vi "ImportExcelValues.vi"(8 "error in (no error)":errorcluster, 9 "List In":refnum<class "List.lvclass">, 10 "ExcelPath":path, 11 "Excel in":refnum<class "Excel.lvclass">) -> (0 "error out":errorcluster, 2 "Sheets":refnum<class "List.lvclass">[](array[class]), 3 "Excel out":refnum<class "Excel.lvclass">)   [LabVIEW 2015, in "Excel.lvclass"]
uses:
  Excel.lvclass
  _list/List.lvclass
  Excel.lvclass/Excel.ctl
  Read_Excel_Values.llb/GetXL_CellValues_2D_String.vi
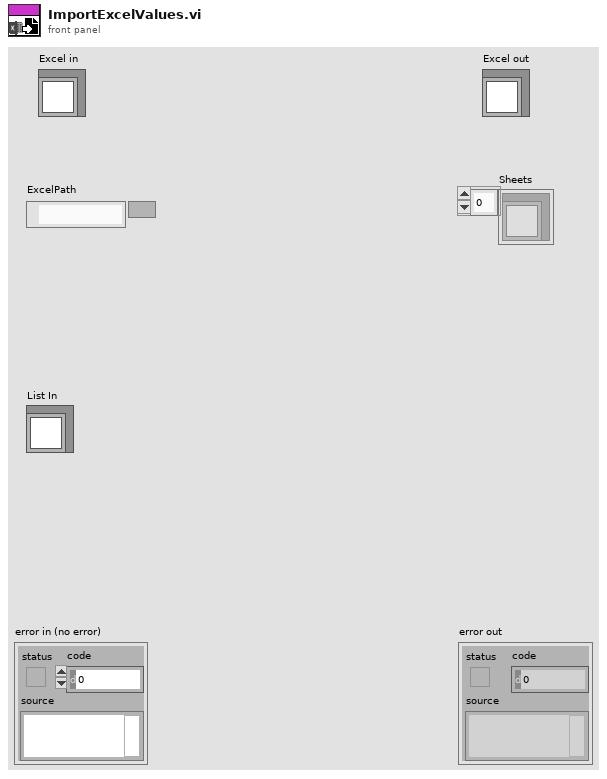
[diagram p1: front panel]
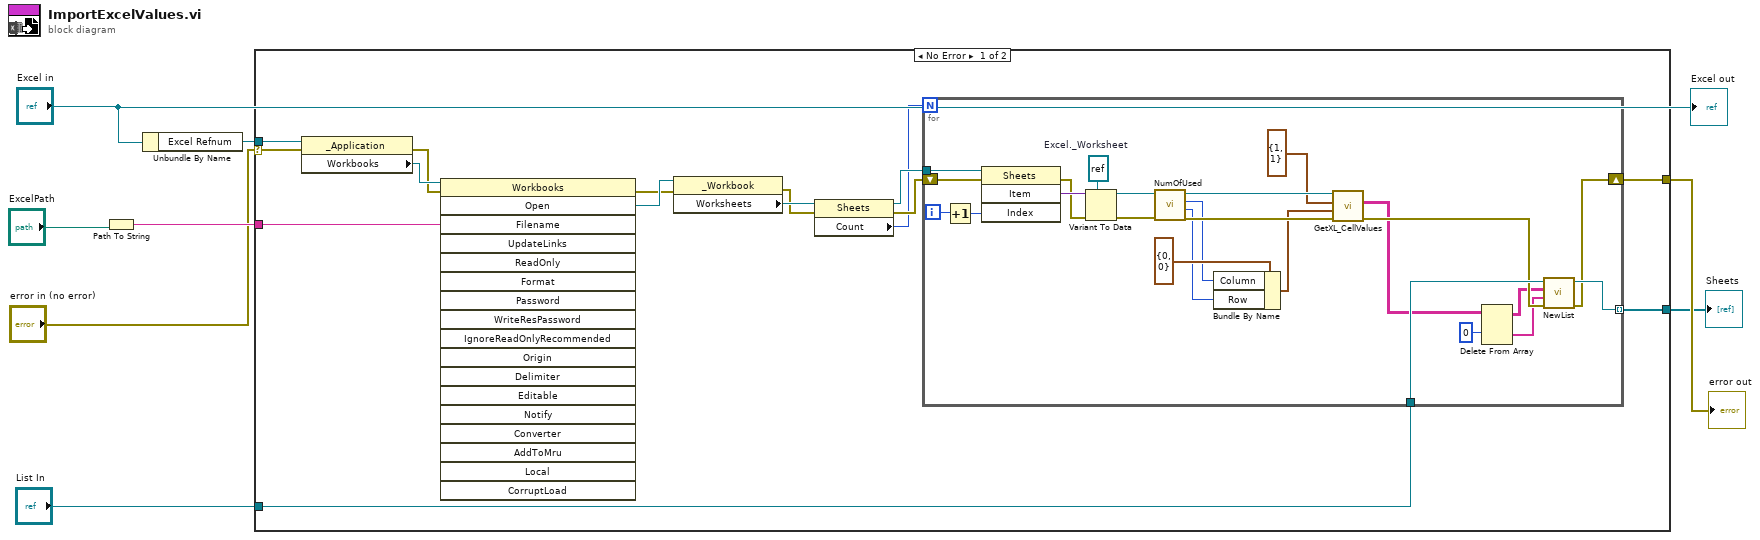
[diagram p0: block diagram]
diagram:
  n1 = Path To String(path="ExcelPath") -> (string=w6:string)
  n2 = Unbundle By Name("Excel in") -> ("Excel Refnum"=w8:refnum<k7>)
  n3 = case shown="No Error" "error in (no error)" {
    selector: "error in (no error)" -> [w16 w48]
    tunnel: w8 -> [w23 _]
    tunnel: w6 -> [w21 _]
    tunnel: [w11 w48] -> w5
    tunnel: [w10 _] -> w2
    tunnel: "List In" -> [w9 _]
    frame No Error {
      n4 = property class="_Application"(reference=w23, error in=w16) -> (error out=w15:errorcluster, "Workbooks"=w22:refnum<k7>)  [unwired: 1 out]
      n5 = invoke class="Workbooks" method="Open"(reference=w22, error in=w15, "Filename"=w21) -> (error out=w14:errorcluster, "Open"=w20:refnum<k7>)  [unwired: 15 in, 16 out]
      n6 = property class="_Workbook"(reference=w20, error in=w14) -> (error out=w13:errorcluster, "Worksheets"=w19:refnum<k7>)  [unwired: 1 out]
      n7 = property class="Sheets"(reference=w19, error in=w13) -> (reference out=w18:refnum<k7>, error out=w17:errorcluster, "Count"=w12:i32)
      n8 = for {
        N: w12 -> [_]
        tunnel: w18 -> [w47]
        shift-right: [w24] -> w11
        shift-left: w17 -> [w46]
        tunnel: [w25] -> w10 mode=indexing
        tunnel: w9 -> [w30]
        i -> [w33]
        w45 = refnum<k7> refnum  # Excel._Worksheet
        n9 = Increment(x=w33) -> (x+1=w32:i32)
        n10 = invoke class="Sheets" method="Item"(reference=w47, error in=w46, "Index"=w32) -> (error out=w34:errorcluster, "Item"=w44:variant)  [unwired: 1 in, 2 out]
        n11 = Variant To Data(error in=w34, type=w45, Variant=w44) -> (data=w43:refnum<k7>, error out=w42:errorcluster)
        n12 = call "NumOfUsed.vi"("error in (no error)"=w42, "worksheet_Refnum"=w43) -> ("error out"=w40:errorcluster, "Rows(0)"=w36:i32, "Columns(0)"=w37:i32, "worksheet_Refnum"=w41:refnum<k7>)  [unwired: 6 in]
        n13 = Bundle By Name(cluster=cluster{"Column":i32, "Row":i32} {"Column"=0, "Row"=0} ("End"), "Column"=w37, "Row"=w36) -> (w35:cluster{"Column":i32, "Row":i32})
        n14 = call-poly "GetXL_CellValues.vi"("error in"=w40, "End"=w35, "Start"=cluster{"Column":i32, "Row":i32} {"Column"=1, "Row"=1}, "worksheet_Refnum"=w41) -> ("error out"=w29:errorcluster, "data"=w28:string[][])  [unwired: 5 in, 1 out]
        n15 = Delete From Array(array=w28, index (row)=0) -> (deleted portion=w27:string[], array with subset deleted=w26:string[][])  [unwired: 2 in]
        n16 = call "NewList.vi"("error in (no error)"=w29, "Titles"=w27, "Contents"=w26, "List In"=w30) -> ("error out"=w24:errorcluster, "List out"=w25:refnum<class "List.lvclass">)  [unwired: 6 in]
      }
    }
    frame Error {
    }
  }
  "error out" <- w5
  "Sheets" <- w2
  "Excel out" <- "Excel in"
